vi "Insight_Dialog_Save_Laser_Parameters_Path.vi"(11 "Path":path) -> (1 "Canceled?":bool, 3 "Path":path)   [LabVIEW 2011]
doc: "Insight Photonic Solutions\n\nThis VI provides a dialog box for the Path to the Save Laser Parameters directory.\n\nver 1.0 - original release"
panel:
  in  "Cancel":bool
  in  "OK":bool
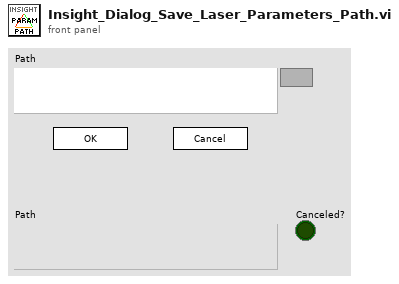
[diagram p1: front panel]
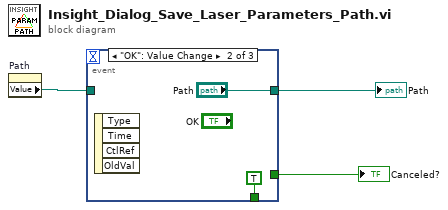
[diagram p0: block diagram]
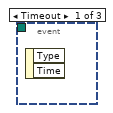
[diagram p2: hidden frame]
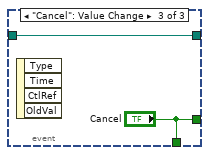
[diagram p3: hidden frame]
diagram:
  n1 = property on="Path" class="Path"() -> ("Value"=w3:path)  [unwired: 2 in, 2 out]
  n2 = event shown="[1] \"OK\": Value Change" {
    selector: _ -> [_ _ _]
    dyn-events: _ -> [_ _ _]
    timeout: _ -> [_ _ _]
    tunnel: [_ "Path" w7] -> w2
    tunnel: [_ TRUE ("Cancel") "Cancel"] -> _
    tunnel: w3 -> [_ _ w7]
    tunnel: [_ _ "Cancel"] -> w1
    event Timeout {
      n3 = event-data() -> ()  [unwired: 1 in, 2 out]
    }
    event "OK": Value Change {
      n4 = event-data() -> ()  [unwired: 1 in, 4 out]
    }
    event "Cancel": Value Change {
      n5 = event-data() -> ()  [unwired: 1 in, 4 out]
    }
  }
  "Path" <- w2
  "Canceled?" <- w1
